vi "Read Data Titles.vi"(8 "error in (no error)":errorcluster, 11 "LakeShore370 in":refnum<class "LakeShore370_device.lvclass">) -> (0 "error out":errorcluster, 2 "Data titles":string[](array[string])=["LS370_R (Ohm)"], 3 "LakeShore370 out":refnum<class "LakeShore370_device.lvclass">)   [LabVIEW 2015, in "LakeShore370_device.lvclass"]
uses:
  LakeShore370_device.lvclass
  LakeSore370 Front Panel Data.ctl
  LakeShore370 Heater Ranges.ctl
  Neocera/Neocera Set Point Aproach.ctl
  OO Devices/Device/Read Controls Snapshot.vi
  OO Devices/Device/Read Control Panel Loaded.vi
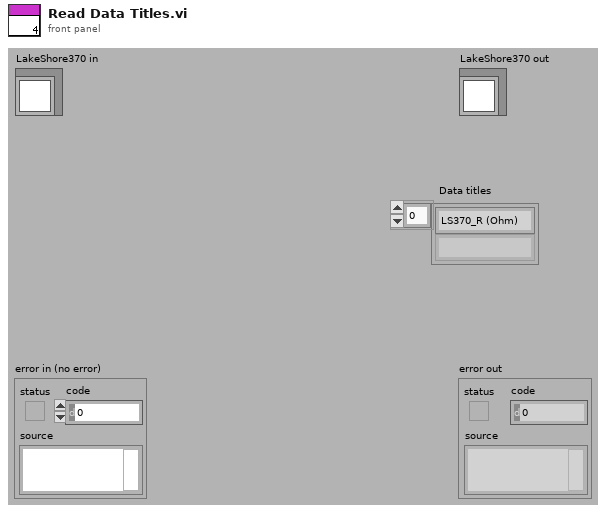
[diagram p1: front panel]
types:
  T1 = typedef "LakeSore370 Front Panel Data.ctl" = cluster{"Channels to scan":i32[], "Scan settling, s":dbl, "Read temperature":bool, "Set point":dbl, "Heater range":T2, "Approach":T3, "Ramp rate, K/min":dbl, "Read heater":bool}
  T2 = typedef "LakeShore370 Heater Ranges.ctl" = enum16{"Off", "31.6uA", "100uA", "316uA", "1mA", "3.16uA", "10mA", "31.6mA", "100mA"}
  T3 = typedef "Neocera Set Point Aproach.ctl" = enum16{"Instant", "Ramp"}
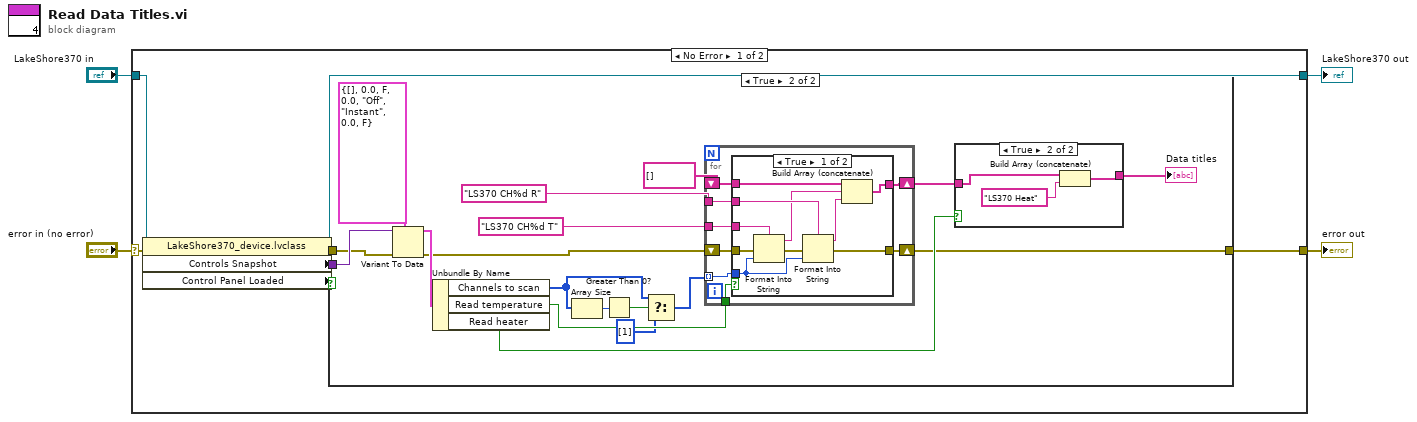
[diagram p0: block diagram]
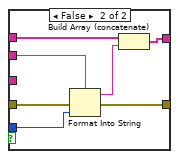
[diagram p4: hidden frame]
diagram:
  n1 = case shown="No Error" "error in (no error)" {
    selector: "error in (no error)" -> [w8 w61]
    tunnel: [w5 w61] -> w3
    tunnel: [w6 w60] -> w1
    tunnel: "LakeShore370 in" -> [w7 w60]
    frame No Error {
      n2 = property class="LakeShore370_device.lvclass"(reference=w7, error in=w8) -> (reference out=w6:refnum<class "LakeShore370_device.lvclass">, error out=w9:errorcluster, "Controls Snapshot"=w10:variant, "Control Panel Loaded"=w11:bool)
      n3 = case shown="True" w11 {
        tunnel: w10 -> [_ w30]
        tunnel: w9 -> [w12 w29]
        tunnel: [w12 w13] -> w5
        frame False {
        }
        frame True {
          n4 = Variant To Data(error in=w29, type=T1 {"Channels to scan"=[], "Scan settling, s"=0.0, "Read temperature"=FALSE, "Set point"=0.0, "Heater range"=enum."Off", "Approach"=enum."Instant", "Ramp rate, K/min"=0.0, "Read heater"=FALSE} ("Data"), Variant=w30) -> (data=w27:T1, error out=w25:errorcluster)
          n5 = Unbundle By Name(w27) -> ("Channels to scan"=w19:i32[], "Read temperature"=w23:bool, "Read heater"=w16:bool)
          n6 = Array Size(array=w19) -> (size(s)=w26:i32)
          n7 = Greater Than 0?(x=w26) -> (x > 0?=w20:bool)
          n8 = Select(t=w19, s=w20, f=i32[] [1]) -> (s? t:f=w18:i32[])
          n9 = for {
            tunnel: w18 -> [w41] mode=indexing
            tunnel: "LS370 CH%d R" -> [w42]
            shift-right: [w39] -> w13
            shift-left: w25 -> [w40]
            tunnel: w23 -> [w38]
            tunnel: "LS370 CH%d T" -> [w37]
            shift-right: [w36] -> w15
            shift-left: string[] [] -> [w35]
            n10 = case shown="True" w38 {
              tunnel: w42 -> [w52 w59]
              tunnel: w41 -> [w48 w57]
              tunnel: w40 -> [w50 w53]
              tunnel: [w51 w58] -> w39
              tunnel: w37 -> [w47 _]
              tunnel: [w44 w55] -> w36
              tunnel: w35 -> [w43 w54]
              frame True {
                n11 = Format Into String(format string=w47, error in=w50, w48) -> (resulting string=w45:string, error out=w49:errorcluster)  [unwired: 1 in]
                n12 = Format Into String(format string=w52, error in=w49, w48) -> (resulting string=w46:string, error out=w51:errorcluster)  [unwired: 1 in]
                n13 = Build Array (concatenate)(w43, w45, w46) -> (w44:string[])
              }
              frame False {
                n14 = Format Into String(format string=w59, error in=w53, w57) -> (resulting string=w56:string, error out=w58:errorcluster)  [unwired: 1 in]
                n15 = Build Array (concatenate)(w54, w56) -> (w55:string[])
              }
            }
          }
          n16 = case shown="True" w16 {
            tunnel: w15 -> [w31 w34]
            tunnel: [w31 w32] -> w14
            frame False {
            }
            frame True {
              n17 = Build Array (concatenate)(w34, "LS370 Heat") -> (w32:string[])
            }
          }
          "Data titles" <- w14
        }
      }
    }
    frame Error {
    }
  }
  "error out" <- w3
  "LakeShore370 out" <- w1
